vi "Write Class Images.vi"(8 "error in (no error)":errorcluster, 10 "Class Images":cluster{"Class Name":string, "Image":T1}[](array[cluster]), 11 "Editor in":refnum<class "Editor.lvclass">) -> (0 "error out":errorcluster, 3 "Editor out":refnum<class "Editor.lvclass">)   [LabVIEW 2015, in "Editor.lvclass"]
uses:
  Editor.lvclass
  <vilib>/picture/picture.llb/imagedata.ctl
  Editor.lvclass/Editor.ctl
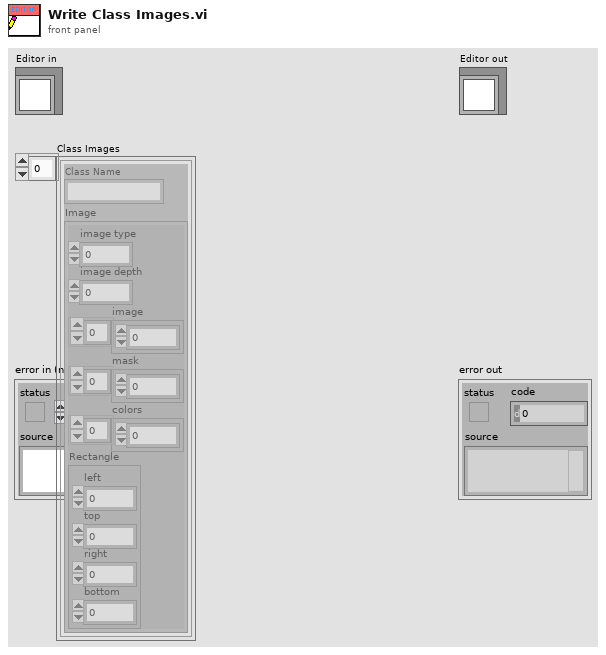
[diagram p1: front panel]
types:
  T1 = typedef "imagedata.ctl" = cluster{"image type":i32, "image depth":i32, "image":u8[], "mask":u8[], "colors":u32[], "Rectangle":cluster{"left":i16, "top":i16, "right":i16, "bottom":i16}}
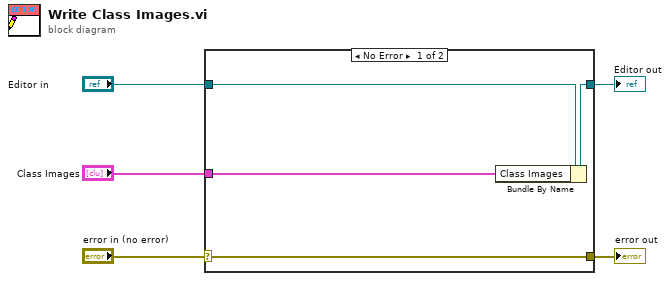
[diagram p0: block diagram]
diagram:
  n1 = case shown="No Error" "error in (no error)" {
    selector: "error in (no error)" -> [w9 w10]
    tunnel: [w9 w10] -> w4
    tunnel: [w7 w11] -> w2
    tunnel: "Editor in" -> [w8 w11]
    tunnel: "Class Images" -> [w6 _]
    frame No Error {
      n2 = Bundle By Name(cluster=w8, "Class Images"=w6) -> (w7:refnum<class "Editor.lvclass">)
    }
    frame Error {
    }
  }
  "error out" <- w4
  "Editor out" <- w2
